vi "Configure Noise Figure.vi"(0 "VISA resource name":refnum<visa-resource-name>, 1 "Sweep Count (11)":dbl=11.0 format="%^#_6g", 5 "ENR Mode (0: Table)":i32(ring) items=["Table", "Spot"], 7 "Average Count (0)":dbl format="%^#_6g", 9 "Resolution Bandwidth (0 Hz)":dbl format="%^#_6g", 11 "error in (no error)":errorcluster, 12 "Enable Internal Preamp (Enabled)":bool=TRUE) -> (4 "VISA resource name out":refnum<visa-resource-name>, 15 "error out":errorcluster)   [LabVIEW 2014, in "Agilent ESA PSA Series.lvlib"]
doc: "Configures the Noise Figure measurement of the Noise Figure personality.\n\n<B>Note:</B> \n\nThis VI is only valid in Noise Figure personality. Use <B>Switch Personality</B> VI to switch to Noise Figure before calling this VI."
uses:
  Agilent ESA PSA Series.lvlib
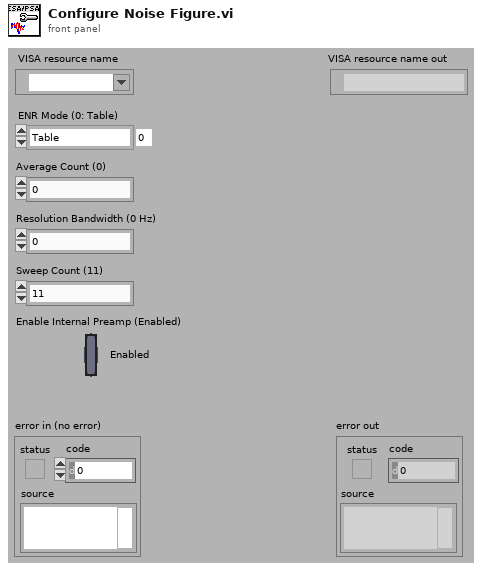
[diagram p1: front panel]
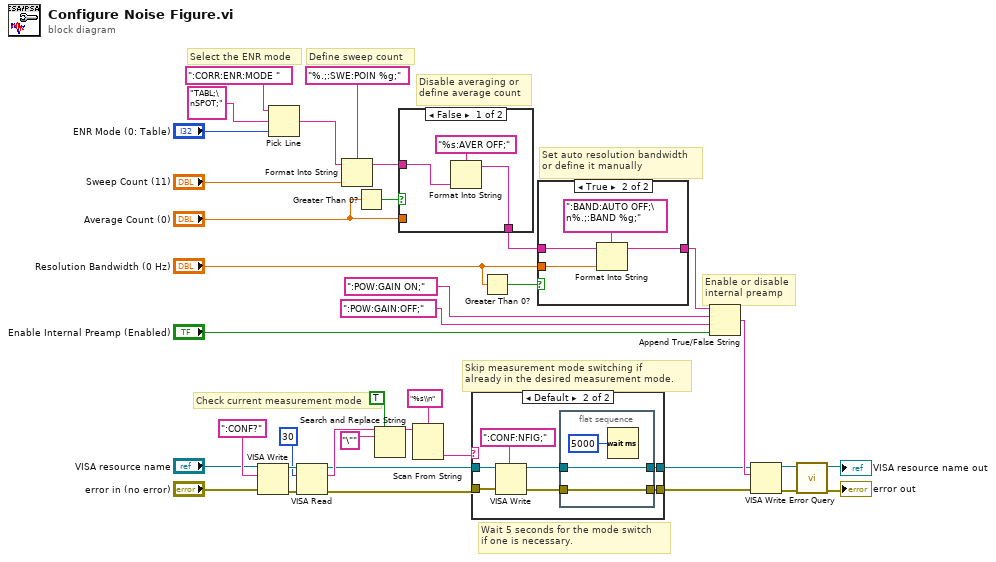
[diagram p0: block diagram]
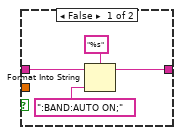
[diagram p3: hidden frame]
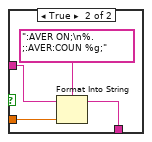
[diagram p4: hidden frame]
diagram:
  # "Wait 5 seconds for the mode switch\nif one is necessary."
  # "Skip measurement mode switching if\nalready in the desired measurement mode."
  # "Check current measurement mode"
  # "Enable or disable\ninternal preamp"
  # "Set auto resolution bandwidth\nor define it manually"
  # "Disable averaging or\ndefine average count"
  # "Define sweep count"
  # "Select the ENR mode"
  n1 = VISA Write(VISA resource name="VISA resource name", write buffer=":CONF?", error in (no error)="error in (no error)") -> (VISA resource name out=w15:refnum<visa-resource-name>, error out=w16:errorcluster)  [unwired: 1 out]
  n2 = Pick Line(string ("")=":CORR:ENR:MODE ", multi-line string="TABL;\nSPOT;", line index="ENR Mode (0: Table)") -> (output string=w30:string)
  n3 = VISA Read(VISA resource name=w15, byte count=u32 30, error in (no error)=w16) -> (VISA resource name out=w7:refnum<visa-resource-name>, read buffer=w8:string, error out=w6:errorcluster)  [unwired: 1 out]
  n4 = Format Into String(format string="%.;:SWE:POIN %g;", initial string=w30, "Sweep Count (11)") -> (resulting string=w27:string)  [unwired: 1 in, 1 out]
  n5 = Greater Than 0?(x="Average Count (0)") -> (x > 0?=w26:bool)
  n6 = Search and Replace String(replace all?=TRUE ("replace all? (F)"), input string=w8, search string="\"") -> (result string=w11:string)  [unwired: 5 in, 3 out]
  n7 = case shown="False" w26 {
    tunnel: "Average Count (0)" -> [_ w44]
    tunnel: w27 -> [w39 w43]
    tunnel: [w38 w41] -> w24
    frame False {
      n8 = Format Into String(format string="%s:AVER OFF;", w39) -> (resulting string=w38:string)  [unwired: 2 in, 1 out]
    }
    frame True {
      n9 = Format Into String(format string=":AVER ON;\n%.;:AVER:COUN %g;", initial string=w43, w44) -> (resulting string=w41:string)  [unwired: 1 in, 1 out]
    }
  }
  n10 = Scan From String(format string="%s\\n", input string=w11) -> (output 1=w9:string)  [unwired: 3 in, 3 out]
  n11 = case shown="Default" w9 {
    tunnel: w7 -> [w46 w53]
    tunnel: w6 -> [w45 w52]
    tunnel: [w46 w48] -> w2
    tunnel: [w45 w47] -> w1
    frame "NFIG", "NFIGure" {
    }
    frame Default {
      n12 = VISA Write(VISA resource name=w53, write buffer=":CONF:NFIG;", error in (no error)=w52) -> (VISA resource name out=w50:refnum<visa-resource-name>, error out=w49:errorcluster)  [unwired: 1 out]
      n13 = flat-sequence {
        tunnel: w50 -> [w56]
        tunnel: w49 -> [w55]
        tunnel: [w56] -> w48
        tunnel: [w55] -> w47
        frame #0 {
          n14 = Wait (ms)(milliseconds to wait=u32 5000) -> ()  [unwired: 1 out]
        }
      }
    }
  }
  n15 = Greater Than 0?(x="Resolution Bandwidth (0 Hz)") -> (x > 0?=w23:bool)
  n16 = case shown="True" w23 {
    tunnel: "Resolution Bandwidth (0 Hz)" -> [_ w64]
    tunnel: w24 -> [w60 w63]
    tunnel: [w57 w61] -> w20
    frame False {
      n17 = Format Into String(format string="%s", initial string=w60, ":BAND:AUTO ON;" ("input 1")) -> (resulting string=w57:string)  [unwired: 1 in, 1 out]
    }
    frame True {
      n18 = Format Into String(format string=":BAND:AUTO OFF;\n%.;:BAND %g;", initial string=w63, w64) -> (resulting string=w61:string)  [unwired: 1 in, 1 out]
    }
  }
  n19 = Append True/False String(1:"Enable Internal Preamp (Enabled)", 2:":POW:GAIN:OFF;" ("false string"), 3:":POW:GAIN ON;" ("true string"), 4:w20) -> (0:w17:string)
  n20 = VISA Write(VISA resource name=w2, write buffer=w17, error in (no error)=w1) -> (VISA resource name out=w35:refnum<visa-resource-name>, error out=w34:errorcluster)  [unwired: 1 out]
  n21 = call "Error Query.vi"("error in (no error)"=w34, "VISA resource name"=w35) -> ("error out"=→"error out":errorcluster, "VISA resource name out"=→"VISA resource name out":refnum<visa-resource-name>)  [unwired: 6 in, 2 out]
